vi "replace cursor - plot ref - V2.vi"(0 "Plot ref in":refnum<vi>, 1 "new X":dbl=nan, 3 "new  Y":dbl=nan, 4 "window IN":T1={"window y"=0.0021014740628288917, "center x"=44850.89441339177, "center y"=2.5658109925320947, "window x"=17480.201988350764} {"window x" format="%#9_9f"; "center y" format="%#9_9f"; "center x" format="%#9_9f"}, 5 "cursor index":i32, 6 "cursor action":T2=enum."write", 7 "label":enum16{"hide", "show x", "show y", "show (x,y)"}(ring), 9 "x-label":string, 11 "y-label":string, 12 "Color Box":u32(colorbox)=327424, 13 "cursor state":T3=enum."boring") -> (14 "Plot ref out":refnum<vi>, 15 "read X":dbl, 18 "read Y":dbl)   [LabVIEW 2017]
uses:
  cursor sate.ctl
  cursor action.ctl
  2Dwindow.ctl
panel:
  in  "action":enum16{"", "read", "write"}(ring)=enum."write"
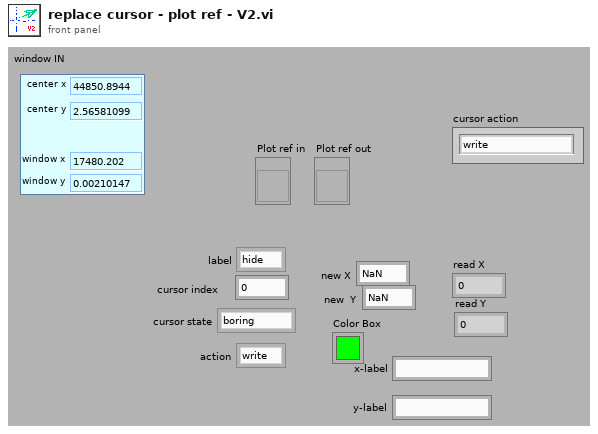
[diagram p1: front panel]
types:
  T1 = typedef "2Dwindow.ctl" = cluster{"window y":dbl, "center x":dbl, "center y":dbl, "window x":dbl}
  T2 = typedef "cursor action.ctl" = enum16{"range", "read", "write", "check", "zoom out", "smart zoom out", "zoom to aspect ratio 1", "zoom to win"}
  T3 = typedef "cursor sate.ctl" = enum16{"normal", "alert", "fuzzy", "interesting", "boring", "colored"}
  T4 = typedef "LVCursorListTypeDef.ctl" = cluster{"Name":string, "Color":u32, "Style":u8, "Point Style":u8, "Name Visible":bool, "Allow Drag":bool, "Cursor Mode":u32, "Plot":i32, "Index":i32, "Position":cluster{"X":dbl, "Y":dbl}, "X Scale":u32, "Y Scale":u32, "Watch Plots":i32[], "Watch All Plots":bool, "Plot Area":i32, "Label Offset":cluster{"X":dbl, "Y":dbl}}[]
  T5 = cluster{"Name":string, "Color":u32, "Style":u8, "Point Style":u8, "Name Visible":bool, "Allow Drag":bool, "Cursor Mode":u32, "Plot":i32, "Index":i32, "Position":cluster{"X":dbl, "Y":dbl}, "X Scale":u32, "Y Scale":u32, "Watch Plots":i32[], "Watch All Plots":bool, "Plot Area":i32, "Label Offset":cluster{"X":dbl, "Y":dbl}}
  T6 = typedef "LVRangeTypeDef.ctl" = cluster{"Minimum":dbl, "Maximum":dbl, "Increment":dbl, "Minor Increment":dbl, "Start":dbl}
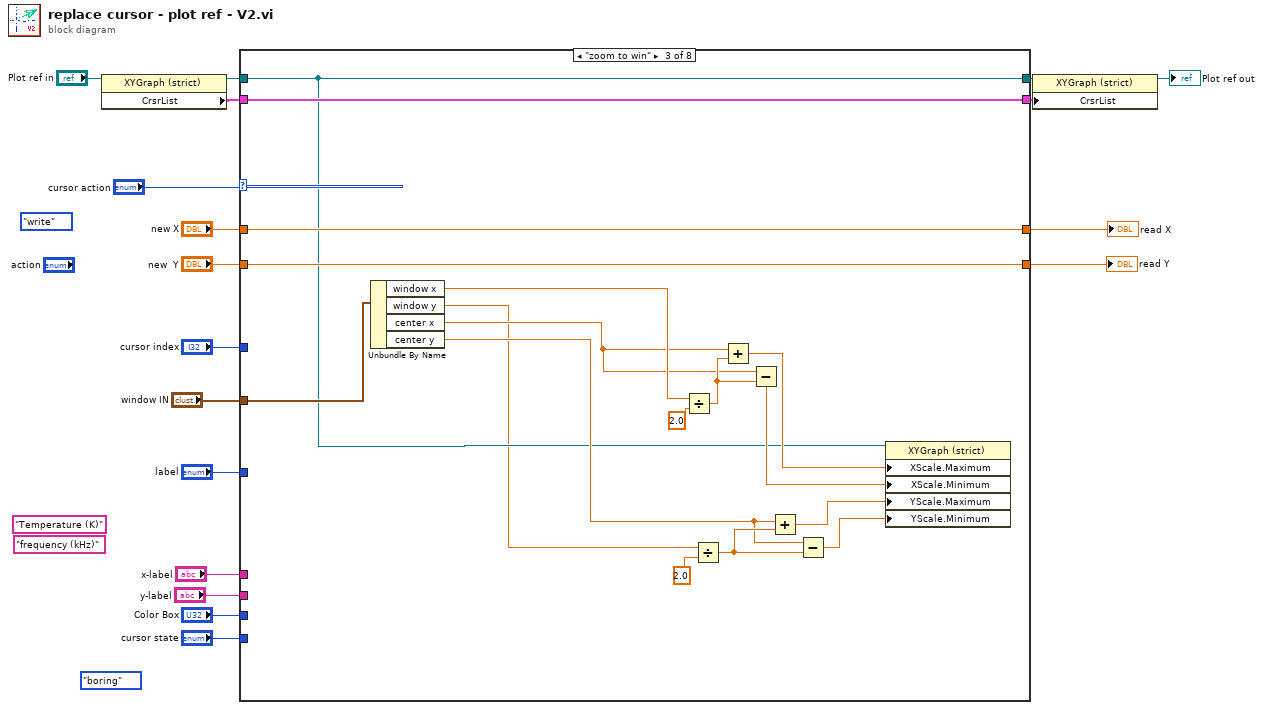
[diagram p0: block diagram]
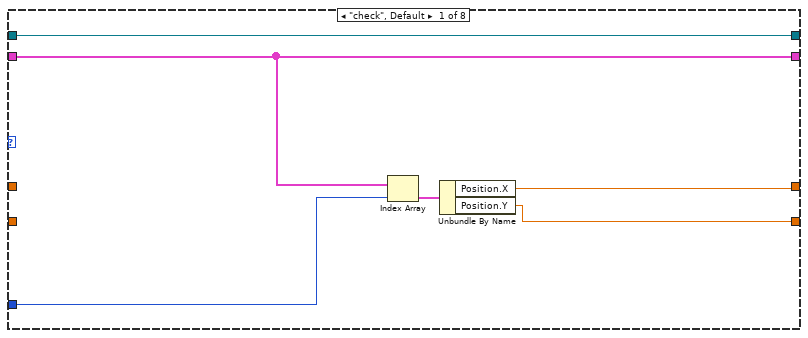
[diagram p2: hidden frame]
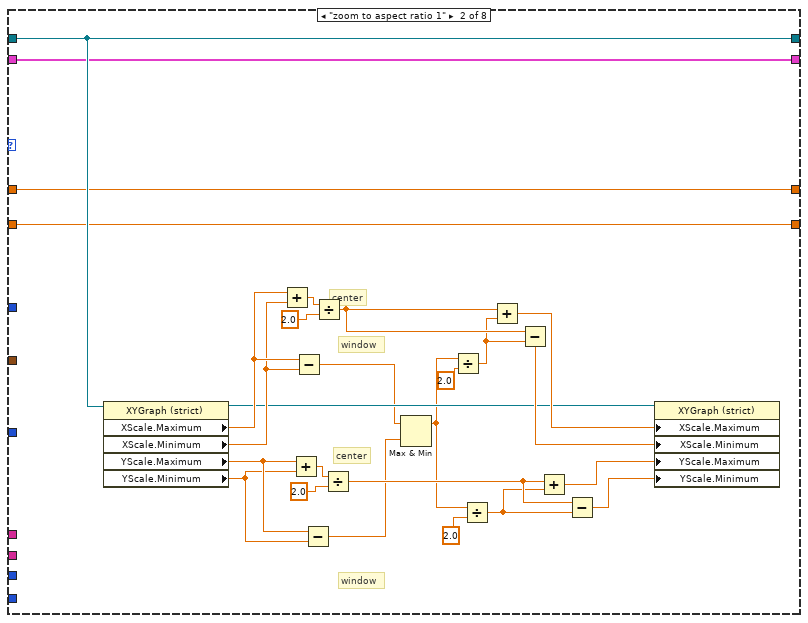
[diagram p3: hidden frame]
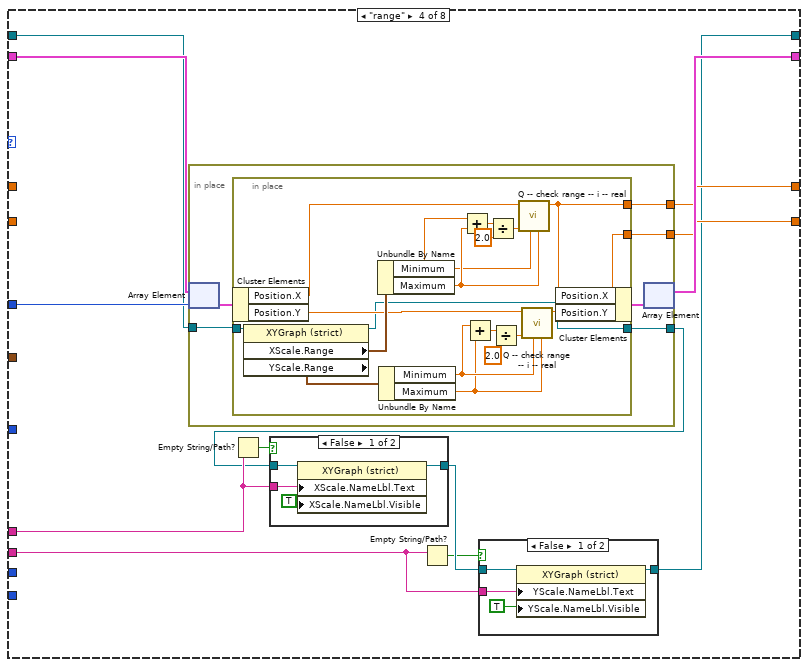
[diagram p4: hidden frame]
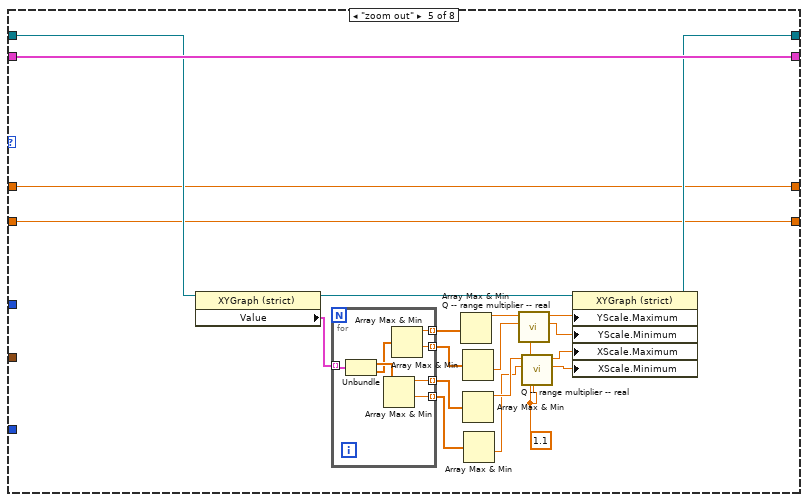
[diagram p7: hidden frame]
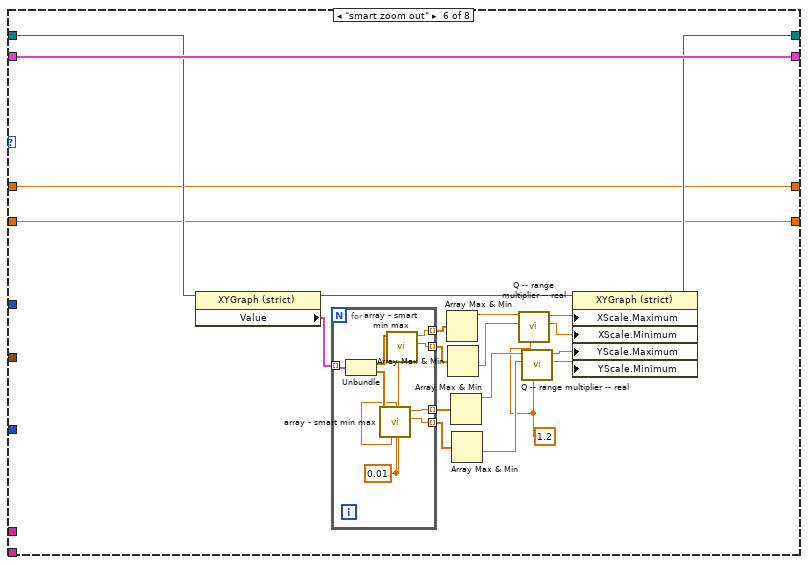
[diagram p8: hidden frame]
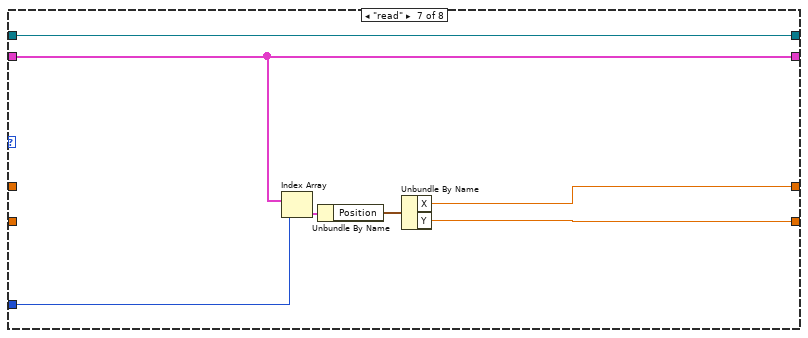
[diagram p9: hidden frame]
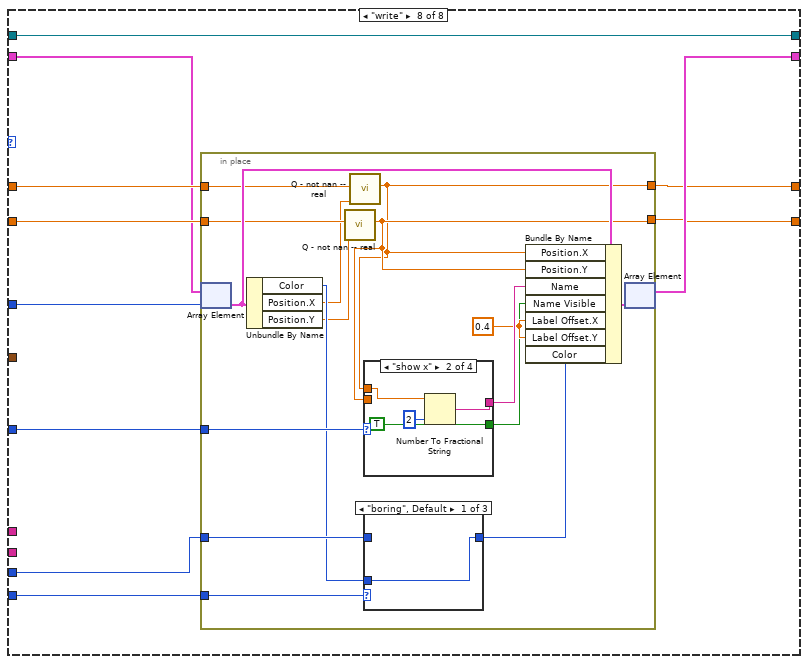
[diagram p10: hidden frame]
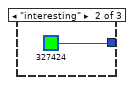
[diagram p11: hidden frame]
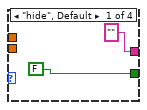
[diagram p13: hidden frame]
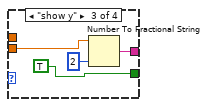
[diagram p14: hidden frame]
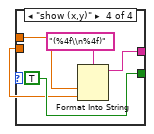
[diagram p15: hidden frame]
diagram:
  (unwired) cursor_sate."boring" ("cursor state")
  (unwired) "frequency (kHz)"
  (unwired) "Temperature (K)"
  (unwired) cursor_action."write" ("cursor action")
  n1 = property on="Property Node" class="XYGraph (strict)"(reference="Plot ref in") -> (reference out=w5:refnum<vi>, "CrsrList"=w13:T4)  [unwired: 1 in, 1 out]
  n2 = case shown="\"zoom to win\"" "cursor action" {
    tunnel: "cursor index" -> [w22 _ _ w78 _ _ w175 w183]
    tunnel: w13 -> [w23 w27 w59 w80 w134 w161 w173 w185]
    tunnel: "new  Y" -> [_ w25 w57 _ w129 w156 _ w186]
    tunnel: "new X" -> [_ w26 w58 _ w130 w157 _ w187]
    tunnel: [w20 w26 w58 w77 w130 w157 w172 w182] -> w15
    tunnel: [w19 w25 w57 w76 w129 w156 w171 w181] -> w14
    tunnel: "label" -> [_ _ _ _ _ _ _ w180]
    tunnel: "Color Box" -> [_ _ _ _ _ _ _ w179]
    tunnel: "cursor state" -> [_ _ _ _ _ _ _ w178]
    tunnel: [w24 w28 w54 w68 w131 w158 w170 w177] -> w6
    tunnel: w5 -> [w24 w28 w54 w75 w133 w160 w170 w177]
    tunnel: "x-label" -> [_ _ _ w73 _ _ _ _]
    tunnel: "y-label" -> [_ _ _ w70 _ _ _ _]
    tunnel: [w23 w27 w59 w79 w134 w161 w173 w184] -> w2
    tunnel: "window IN" -> [_ _ w56 _ _ _ _ _]
    frame "check", Default {
      n3 = Index Array(array=w23, index=w22) -> (element=w21:T5)
      n4 = Unbundle By Name(w21) -> ("Position.X"=w20:dbl, "Position.Y"=w19:dbl)
    }
    frame "zoom to aspect ratio 1" {
      # "window"
      # "center"
      # "window"
      # "center"
      n5 = property on="Property Node" class="XYGraph (strict)"(reference=w28) -> (reference out=w41:refnum<vi>, "XScale.Maximum"=w48:dbl, "XScale.Minimum"=w47:dbl, "YScale.Maximum"=w36:dbl, "YScale.Minimum"=w35:dbl)  [unwired: 1 in, 1 out]
      n6 = Add(x=w48, y=w47) -> (x+y=w50:dbl)
      n7 = Add(x=w36, y=w35) -> (x+y=w40:dbl)
      n8 = Subtract(x=w48, y=w47) -> (x-y=w34:dbl)
      n9 = Subtract(x=w36, y=w35) -> (x-y=w33:dbl)
      n10 = Divide(x=w50, y=2.0) -> (x/y=w44:dbl)
      n11 = Divide(x=w40, y=2.0) -> (x/y=w38:dbl)
      n12 = Max & Min(x=w34, y=w33) -> (max(x,y)=w31:dbl)  [unwired: 1 out]
      n13 = Divide(x=w31, y=2.0) -> (x/y=w43:dbl)
      n14 = Divide(x=w31, y=2.0) -> (x/y=w37:dbl)
      n15 = Add(x=w44, y=w43) -> (x+y=w45:dbl)
      n16 = Subtract(x=w44, y=w43) -> (x-y=w42:dbl)
      n17 = Add(x=w38, y=w37) -> (x+y=w30:dbl)
      n18 = Subtract(x=w38, y=w37) -> (x-y=w29:dbl)
      n19 = property on="Property Node" class="XYGraph (strict)"(reference=w41, "XScale.Maximum"=w45, "XScale.Minimum"=w42, "YScale.Maximum"=w30, "YScale.Minimum"=w29) -> ()  [unwired: 1 in, 2 out]
    }
    frame "zoom to win" {
      n20 = Unbundle By Name(w56) -> ("window x"=w53:dbl, "window y"=w51:dbl, "center x"=w52:dbl, "center y"=w55:dbl)
      n21 = Divide(x=w53, y=2.0) -> (x/y=w65:dbl)
      n22 = Divide(x=w51, y=2.0) -> (x/y=w63:dbl)
      n23 = Add(x=w52, y=w65) -> (x+y=w66:dbl)
      n24 = Subtract(x=w52, y=w65) -> (x-y=w64:dbl)
      n25 = Add(x=w55, y=w63) -> (x+y=w61:dbl)
      n26 = Subtract(x=w55, y=w63) -> (x-y=w60:dbl)
      n27 = property on="Property Node" class="XYGraph (strict)"(reference=w54, "XScale.Maximum"=w66, "XScale.Minimum"=w64, "YScale.Maximum"=w61, "YScale.Minimum"=w60) -> ()  [unwired: 1 in, 2 out]
    }
    frame "range" {
      n28 = in-place {
        in-place-border: w75 -> [w94]
        in-place-border: [w93] -> w77
        in-place-border: [w92] -> w76
        in-place-border: [w91] -> w69
        n29 = in-place-array #1(w80, w78) -> (w96:T5)
        n30 = in-place {
          in-place-border: w94 -> [w102]
          in-place-border: [w99] -> w93
          in-place-border: [w98] -> w92
          in-place-border: [w97] -> w91
          n31 = in-place-cluster #2(w96) -> ("Position.X"=w101:dbl, "Position.Y"=w100:dbl)
          n32 = property on="Property Node" class="XYGraph (strict)"(reference=w102) -> (reference out=w97:refnum<vi>, "XScale.Range"=w103:T6, "YScale.Range"=w104:T6)  [unwired: 1 in, 1 out]
          n33 = Unbundle By Name(w103) -> ("Minimum"=w105:dbl, "Maximum"=w106:dbl)
          n34 = Unbundle By Name(w104) -> ("Minimum"=w114:dbl, "Maximum"=w113:dbl)
          n35 = Add(x=w105, y=w106) -> (x+y=w107:dbl)
          n36 = Add(x=w114, y=w113) -> (x+y=w110:dbl)
          n37 = Divide(x=w107, y=2.0) -> (x/y=w109:dbl)
          n38 = Divide(x=w110, y=2.0) -> (x/y=w112:dbl)
          n39 = call "Q -- check range -- i -- real.vi"("upper"=w106, "lower"=w105, "default"=w109, "number"=w101) -> ("number in range"=w99:dbl)  [unwired: 5 in, 2 out]
          n40 = call "Q -- check range -- i -- real.vi"("upper"=w113, "lower"=w114, "default"=w112, "number"=w100) -> ("number in range"=w98:dbl)  [unwired: 5 in, 2 out]
          n41 = in-place-cluster #2("Position.X"=w99, "Position.Y"=w98) -> (w95:T5)
        }
        n42 = in-place-array #1(w95) -> (w79:T4)  [unwired: 1 out]
      }
      n43 = Empty String/Path?(string/path=w73) -> (empty?=w74:bool)
      n44 = case shown="False" w74 {
        tunnel: w69 -> [w89 w90]
        tunnel: w73 -> [w88 _]
        tunnel: [w87 w90] -> w72
        frame False {
          n45 = property on="Property Node" class="XYGraph (strict)"(reference=w89, "XScale.NameLbl.Text"=w88, "XScale.NameLbl.Visible"=TRUE ("X Scale.Name Label.Visible")) -> (reference out=w87:refnum<vi>)  [unwired: 1 in, 1 out]
        }
        frame True {
        }
      }
      n46 = Empty String/Path?(string/path=w70) -> (empty?=w71:bool)
      n47 = case shown="False" w71 {
        tunnel: w72 -> [w84 w85]
        tunnel: w70 -> [w83 _]
        tunnel: [w82 w85] -> w68
        frame False {
          n48 = property on="Property Node" class="XYGraph (strict)"(reference=w84, "YScale.NameLbl.Text"=w83, "YScale.NameLbl.Visible"=TRUE ("X Scale.Name Label.Visible")) -> (reference out=w82:refnum<vi>)  [unwired: 1 in, 1 out]
        }
        frame True {
        }
      }
    }
    frame "zoom out" {
      w115 = 1.1 ("factor")
      n49 = property on="Property Node" class="XYGraph (strict)"(reference=w133) -> (reference out=w132:refnum<vi>, "Value"=w128:cluster{dbl[], dbl[]}[])  [unwired: 1 in, 1 out]
      n50 = for {
        tunnel: w128 -> [w135] mode=indexing
        tunnel: [w136] -> w124 mode=indexing
        tunnel: [w137] -> w125 mode=indexing
        tunnel: [w138] -> w126 mode=indexing
        tunnel: [w139] -> w127 mode=indexing
        n51 = Unbundle(w135) -> (w141:dbl[], w140:dbl[])
        n52 = Array Max & Min(array=w141) -> (max value=w137:dbl, min value=w136:dbl)  [unwired: 2 out]
        n53 = Array Max & Min(array=w140) -> (max value=w139:dbl, min value=w138:dbl)  [unwired: 2 out]
      }
      n54 = Array Max & Min(array=w127) -> (max value=w119:dbl)  [unwired: 3 out]
      n55 = Array Max & Min(array=w126) -> (min value=w118:dbl)  [unwired: 3 out]
      n56 = Array Max & Min(array=w125) -> (max value=w117:dbl)  [unwired: 3 out]
      n57 = Array Max & Min(array=w124) -> (min value=w116:dbl)  [unwired: 3 out]
      n58 = call "Q -- range multiplier -- real.vi"("factor"=w115, "lower"=w118, "upper"=w119) -> ("lower OUT"=w120:dbl, "upper OUT"=w121:dbl)  [unwired: 5 in, 2 out]
      n59 = call "Q -- range multiplier -- real.vi"("factor"=w115, "lower"=w116, "upper"=w117) -> ("lower OUT"=w122:dbl, "upper OUT"=w123:dbl)  [unwired: 5 in, 2 out]
      n60 = property on="Property Node" class="XYGraph (strict)"(reference=w132, "YScale.Maximum"=w121, "YScale.Minimum"=w120, "XScale.Maximum"=w123, "XScale.Minimum"=w122) -> (reference out=w131:refnum<vi>)  [unwired: 1 in, 1 out]
    }
    frame "smart zoom out" {
      w142 = 1.2 ("factor")
      n61 = property on="Property Node" class="XYGraph (strict)"(reference=w160) -> (reference out=w159:refnum<vi>, "Value"=w155:cluster{dbl[], dbl[]}[])  [unwired: 1 in, 1 out]
      n62 = for {
        tunnel: w155 -> [w167] mode=indexing
        tunnel: [w166] -> w148 mode=indexing
        tunnel: [w168] -> w145 mode=indexing
        tunnel: [w163] -> w144 mode=indexing
        tunnel: [w169] -> w150 mode=indexing
        w162 = 0.01 ("median range")
        n63 = Unbundle(w167) -> (w165:dbl[], w164:dbl[])
        n64 = call "array - smart min max.vi"("median range"=w162, "x"=w164) -> ("min"=w166:dbl, "max"=w168:dbl)  [unwired: 8 in]
        n65 = call "array - smart min max.vi"("median range"=w162, "x"=w165) -> ("min"=w163:dbl, "max"=w169:dbl)  [unwired: 8 in]
      }
      n66 = Array Max & Min(array=w150) -> (max value=w149:dbl)  [unwired: 3 out]
      n67 = Array Max & Min(array=w144) -> (min value=w143:dbl)  [unwired: 3 out]
      n68 = Array Max & Min(array=w145) -> (max value=w146:dbl)  [unwired: 3 out]
      n69 = Array Max & Min(array=w148) -> (min value=w147:dbl)  [unwired: 3 out]
      n70 = call "Q -- range multiplier -- real.vi"("factor"=w142, "lower"=w143, "upper"=w149) -> ("lower OUT"=w151:dbl, "upper OUT"=w152:dbl)  [unwired: 5 in, 2 out]
      n71 = call "Q -- range multiplier -- real.vi"("factor"=w142, "lower"=w147, "upper"=w146) -> ("lower OUT"=w153:dbl, "upper OUT"=w154:dbl)  [unwired: 5 in, 2 out]
      n72 = property on="Property Node" class="XYGraph (strict)"(reference=w159, "XScale.Maximum"=w152, "XScale.Minimum"=w151, "YScale.Maximum"=w154, "YScale.Minimum"=w153) -> (reference out=w158:refnum<vi>)  [unwired: 1 in, 1 out]
    }
    frame "read" {
      n73 = Index Array(array=w173, index=w175) -> (element=w176:T5)
      n74 = Unbundle By Name(w176) -> ("Position"=w174:cluster{"X":dbl, "Y":dbl})
      n75 = Unbundle By Name(w174) -> ("X"=w172:dbl, "Y"=w171:dbl)
    }
    frame "write" {
      n76 = in-place {
        in-place-border: w187 -> [w190]
        in-place-border: w186 -> [w193]
        in-place-border: [w189] -> w182
        in-place-border: [w191] -> w181
        in-place-border: w180 -> [w199]
        in-place-border: w179 -> [w196]
        in-place-border: w178 -> [w197]
        w200 = 0.4 ("Label Offset.X")
        n77 = in-place-array #3(w185, w183) -> (w203:T5)
        n78 = Unbundle By Name(w203) -> ("Color"=w194:u32, "Position.X"=w188:dbl, "Position.Y"=w192:dbl)
        n79 = call "Q - not nan -- real.vi"("default"=w192, "Numeric"=w193) -> ("out"=w191:dbl)  [unwired: 8 in, 1 out]
        n80 = call "Q - not nan -- real.vi"("default"=w188, "Numeric"=w190) -> ("out"=w189:dbl)  [unwired: 8 in, 1 out]
        n81 = case shown="\"show x\"" w199 {
          tunnel: w189 -> [_ w212 _ w218]
          tunnel: ["" ("format string") w211 w215 w221] -> w202
          tunnel: [FALSE ("Name Visible") TRUE ("Name Visible") TRUE ("Name Visible") TRUE ("Name Visible")] -> w198
          tunnel: w191 -> [_ _ w214 w217]
          frame "hide", Default {
          }
          frame "show x" {
            n82 = Number To Fractional String(number=w212, precision (6)=i16 2) -> (F-format string=w211:string)  [unwired: 2 in]
          }
          frame "show y" {
            n83 = Number To Fractional String(number=w214, precision (6)=i16 2) -> (F-format string=w215:string)  [unwired: 2 in]
          }
          frame "show (x,y)" {
            n84 = Format Into String(format string="(%4f\\n%4f)", w218, w217) -> (resulting string=w221:string)  [unwired: 2 in, 1 out]
          }
        }
        n85 = case shown="\"boring\", Default" w197 {
          tunnel: [w204 u32 327424 ("Color Box") w206] -> w195
          tunnel: w196 -> [_ _ w206]
          tunnel: w194 -> [w204 _ _]
          frame "boring", Default {
          }
          frame "interesting" {
          }
          frame "colored" {
          }
        }
        n86 = Bundle By Name(cluster=w203, "Position.X"=w189, "Position.Y"=w191, "Name"=w202, "Name Visible"=w198, "Label Offset.X"=w200, "Label Offset.Y"=w200, "Color"=w195) -> (w201:T5)
        n87 = in-place-array #3(w201) -> (w184:T4)  [unwired: 1 out]
      }
    }
  }
  "read X" <- w15
  "read Y" <- w14
  n88 = property on="Property Node" class="XYGraph (strict)"(reference=w6, "CrsrList"=w2) -> (reference out=→"Plot ref out":refnum<vi>)  [unwired: 1 in, 1 out]
